vi "Read Device Channel Names.vi"(8 "error in (no error)":errorcluster, 11 "2525 in":refnum<class "2525.lvclass">) -> (0 "error out":errorcluster, 2 "Device Channel Names":string[](array[string]), 3 "2525 out":refnum<class "2525.lvclass">)   [LabVIEW 2019, in "2525.lvlib" / "2525.lvclass"]
uses:
  Library/2525.lvclass
  Library/2525.lvclass/2525.ctl
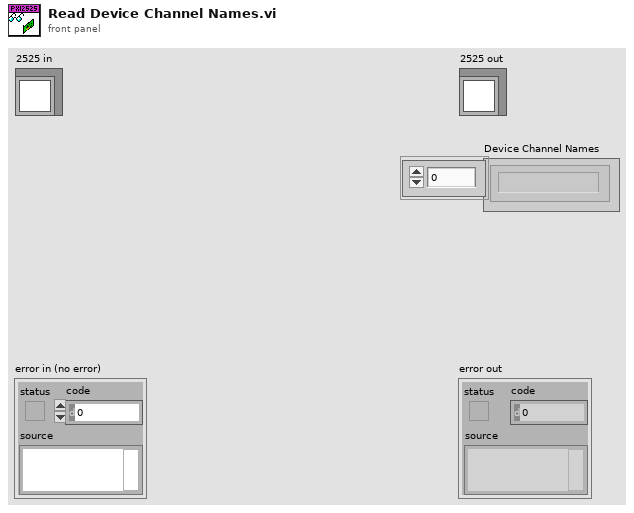
[diagram p1: front panel]
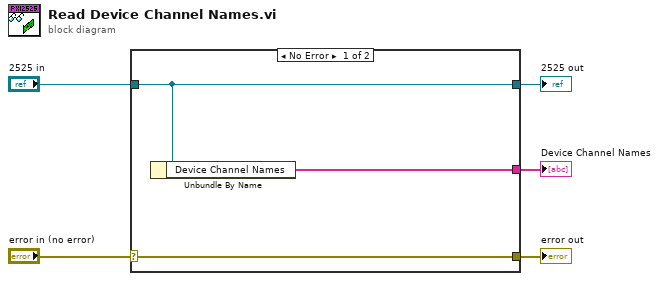
[diagram p0: block diagram]
diagram:
  n1 = case shown="No Error" "error in (no error)" {
    selector: "error in (no error)" -> [w8 w9]
    tunnel: [w8 w9] -> w4
    tunnel: [w7 w10] -> w2
    tunnel: "2525 in" -> [w7 w10]
    tunnel: [w6 _] -> w1
    frame No Error {
      n2 = Unbundle By Name(w7) -> ("Device Channel Names"=w6:string[])
    }
    frame Error {
    }
  }
  "error out" <- w4
  "2525 out" <- w2
  "Device Channel Names" <- w1
